vi "Actor Core.vi"(8 "error in":errorcluster, 11 "CS++DCPwrGui.lvclass":refnum<class "CS++DCPwrGui.lvclass">) -> (0 "Error Out":errorcluster, 3 "Actor out":refnum<class "Actor.lvclass">)   [LabVIEW 2014, in "CS++DCPwrGui.lvlib" / "CS++DCPwrGui.lvclass"]
doc: "(<B>Filename</B>: Actor Framework.lvlib:Actor.lvclass:Actor Core.vi)\n\nReceives messages to the actor, reacts to them, and initiates any error handling that may shut the actor down.\n\nDescendant classes may override this VI to append parallel tasks for the actor to complete while it handles messages. Overrides use the Call Parent Method node."
uses:
  CS++DCPwrGui.lvclass
  <vilib>/ActorFramework/Actor/Actor.lvclass
  CSPP_Core/Actors/CS++BaseActor/CS++BaseActor.lvclass/CS++BaseActor.ctl
  CS++DCPwrChannelData/CS++DCPwrChannelData.lvclass
  CSPP_Core/Actors/CS++GUIActor/CS++GUIActor.lvclass/CS++GUIActor.ctl
  <vilib>/ActorFramework/Actor/Actor.lvclass/Actor.ctl
  <vilib>/ActorFramework/Message Enqueuer/Message Enqueuer.lvclass/Message Enqueuer.ctl
  CSPP_Core/Classes/CS++ProcessVariables/ProcessVariable/PV.lvclass/PV.ctl
  CS++DCPwrChannelData/CS++DCPwrChannelData.lvclass/CS++DCPwrChannelData.ctl
  CS++DCPwr Messages/Configure Voltage Level Msg/Configure Voltage Level Msg.lvclass/Configure Voltage Level Msg.ctl
  CS++DCPwr Messages/Reset Output Protection Msg/Reset Output Protection Msg.lvclass/Reset Output Protection Msg.ctl
  CS++DCPwr Messages/Measure [MSR] Msg/Measure [MSR] Msg.lvclass
  CS++DCPwr Messages/Measure [MSR] Msg/Measure [MSR] Msg.lvclass/Measure [MSR] Msg.ctl
  <vilib>/ActorFramework/Batch Msg/Batch Msg.lvclass/Batch Msg.ctl
  CS++DCPwr Messages/Configure Output Enable Msg/Configure Output Enable Msg.lvclass/Configure Output Enable Msg.ctl
  CS++DCPwr Messages/Configure Desired Output State Msg/Configure Desired Output State Msg.lvclass/Configure Desired Output State Msg.ctl
  CS++DCPwr Messages/Configure Output Range Msg/Configure Output Range Msg.lvclass/Configure Output Range Msg.ctl
  CS++DCPwr Messages/Configure OVP Msg/Configure OVP Msg.lvclass/Configure OVP Msg.ctl
  CS++DCPwr Messages/Configure Current Limit Msg/Configure Current Limit Msg.lvclass/Configure Current Limit Msg.ctl
  CS++DCPwr Messages/Configure Trigger Source [TRG] Msg/Configure Trigger Source [TRG] Msg.lvclass/Configure Trigger Source [TRG] Msg.ctl
  CS++DCPwr Messages/Configure Triggered Current Limit [TRG] Msg/Configure Triggered Current Limit [TRG] Msg.lvclass/Configure Triggered Current Limit [TRG] Msg.ctl
  CS++DCPwr Messages/Configure Triggered Voltage Level [TRG] Msg/Configure Triggered Voltage Level [TRG] Msg.lvclass/Configure Triggered Voltage Level [TRG] Msg.ctl
  CSPP_Core/Actors/CS++BaseActor/Read Object Name.vi
  CSPP_Core/Actors/CS++BaseActor/Read CS++Factory.vi
  CSPP_Core/Classes/CS++ProcessVariables/ProcessVariable/Read Data.vi
  CSPP_Core/Classes/CS++ProcessVariables/ProcessVariable/Read Timestamp.vi
  CSPP_Core/Classes/CS++ProcessVariables/ProcessVariable/Read Name.vi
  CS++DCPwr Messages/Measure [MSR] Msg/Write channel name.vi
  CS++DCPwr Messages/Measure [MSR] Msg/Write measurement type.vi
  <vilib>/ActorFramework/Message Enqueuer/Init from Existing Queue.vi
  <vilib>/ActorFramework/Message Enqueuer/Enqueue.vi
  CSPP_Core/Actors/CS++GUIActor/Read Associated Actor Name.vi
  <vilib>/ActorFramework/Message Priority Queue/Priority Enqueue.vi
  CSPP_Core/Classes/CS++BaseClasses/Factory/CS++Factory.lvclass
  CSPP_Core/Classes/CS++ProcessVariables/ProcessVariable/PV.lvclass
  <vilib>/ActorFramework/Message Enqueuer/Message Enqueuer.lvclass
  <vilib>/ActorFramework/Stop Msg/Stop Msg.lvclass
  CS++DCPwr Messages/Configure Voltage Level Msg/Configure Voltage Level Msg.lvclass
  CS++DCPwr Messages/Reset Output Protection Msg/Reset Output Protection Msg.lvclass
  CS++DCPwr Messages/Initiate [TRG] Msg/Initiate [TRG] Msg.lvclass
  CS++DCPwr Messages/Send Software Trigger [SWT] Msg/Send Software Trigger [SWT] Msg.lvclass
  CS++DCPwr Messages/Abort [TRG] Msg/Abort [TRG] Msg.lvclass
  <vilib>/ActorFramework/Batch Msg/Batch Msg.lvclass
  CS++DCPwr Messages/Configure Output Enable Msg/Configure Output Enable Msg.lvclass
  CS++DCPwr Messages/Configure Desired Output State Msg/Configure Desired Output State Msg.lvclass
  CS++DCPwr Messages/Configure Output Range Msg/Configure Output Range Msg.lvclass
  CS++DCPwr Messages/Configure OVP Msg/Configure OVP Msg.lvclass
  CS++DCPwr Messages/Configure Current Limit Msg/Configure Current Limit Msg.lvclass
  CS++DCPwr Messages/Configure Trigger Source [TRG] Msg/Configure Trigger Source [TRG] Msg.lvclass
  CS++DCPwr Messages/Configure Triggered Current Limit [TRG] Msg/Configure Triggered Current Limit [TRG] Msg.lvclass
  CS++DCPwr Messages/Configure Triggered Voltage Level [TRG] Msg/Configure Triggered Voltage Level [TRG] Msg.lvclass
  CSPP_Core/Actors/CS++DeviceGUIActor/CS++DeviceGUIActor.lvclass
  CSPP_Core/Actors/CS++BaseActor/CS++BaseActor.lvclass
  CSPP_Core/Actors/CS++GUIActor/CS++GUIActor.lvclass
  CSPP_Core/Libraries/Utilities/CS++Utilities.lvlib
panel:
  in  "Tab Control":enum32{"Info", "Configuration", "Output"}(tab)
  out "Associated Actor":string
  out "Driver Revision":string
  out "Firmware Revision":string
  out "Self-Test Result Code":i32
  out "Self-Test Result Message":string
  out "Resource Name":string
  out "Number Of Channels":i32
  in  "Config Index":i32 min=0 step=1
  in  "OVP":T1 {"OVP Limit" format="%^.3g"}
  in  "Current":T2 {"Behavior" items=["Regulate", "Trip"]; "Current Limit" format="%^.3g"}
  in  "Range":cluster{"Range Type":i32, "Range":dbl}={"Range Type"=1, "Range"=0.0} {"Range" format="%^.3g"; "Range Type" items=["Voltage"=1, "Current"=0]}
  in  "Output State":i32(ring) caption="output state (Constant Voltage)" items=["Constant Voltage"=0, "Constant Current"=1, "Unregulated"=4, "Over Voltage"=2, "Over Current"=3]
  in  "Output Enable":bool caption="enabled (true)"
  in  "Trigger":T3 {"Triggered I-Limit" format="%^.6g"; "Triggered U-Level" format="%^.6g"; "Trigger Source" items=["Immediate", "External", "Software", "TTL0", "TTL1", "TTL2", "TTL3", "TTL4", "TTL5", "TTL6", "TTL7", "ECL0", "ECL1", "PXI Star", "RTSI 0", "RTSI 1", "RTSI 2", "RTSI 3", "RTSI 4", "RTSI 5", "RTSI 6"]}
  out "Maximum Limits":T4 {"Max Voltage Level" format="%^.3g"; "Max Current Limit" format="%^.3g"}
  in  "Level":dbl[unit] caption="level (0.0 Volts)" format="%^.6g"
  in  "Channel Index":i32 min=0 step=1
  in  "Reset Output Protection":bool
  in  "Initiate":bool
  in  "Software Trigger":bool
  in  "Abort":bool
  in  "Sense now":bool
  out "Timestamp":timestamp
  out "Measurements":T5(array[cluster]) {"Actual U" format="%.6g"; "Actual I" format="%.6g"}
  in  "Stop Button":bool
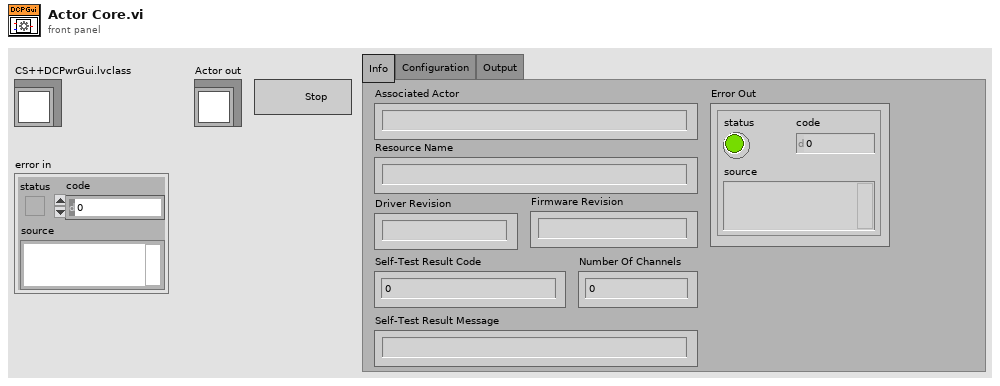
[diagram p1: front panel]
types:
  T1 = cluster{"OVP Enabled":bool, "OVP Limit":dbl[unit]}
  T2 = cluster{"Behavior":i32, "Current Limit":dbl[unit]}
  T3 = cluster{"Trigger Source":i32, "Triggered U-Level":dbl[unit], "Triggered I-Limit":dbl[unit]}
  T4 = cluster{"Max Current Limit":dbl[unit], "Max Voltage Level":dbl[unit]}
  T5 = cluster{"Actual U":dbl[unit], "Actual I":dbl[unit], "In State":bool}[]
  T6 = enum32{"Invalid", "Standard", "Closed", "Hidden", "Minimized", "Maximized"}
  T7 = cluster{"measurement":dbl[unit], "measurement":dbl[unit], "in state":bool}[]
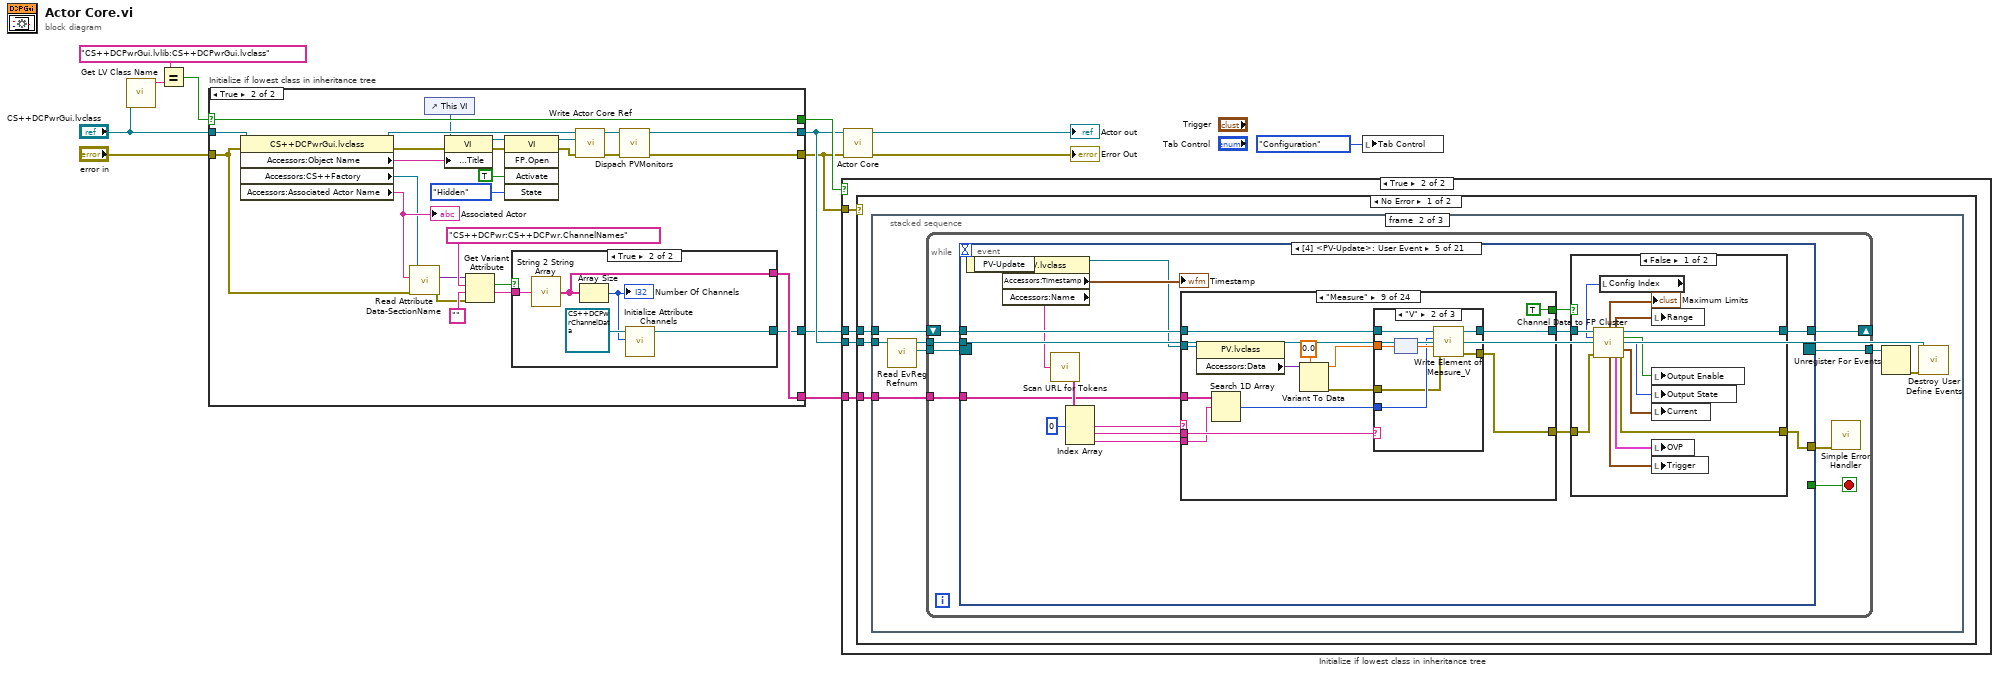
[diagram p0: block diagram]
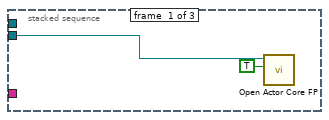
[diagram p5: hidden frame]
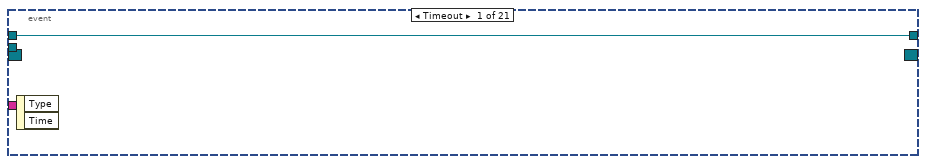
[diagram p6: hidden frame]
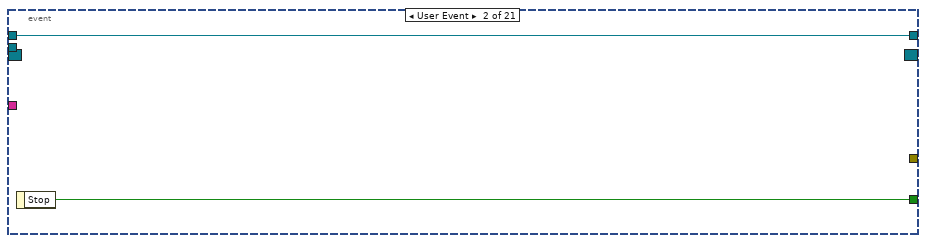
[diagram p7: hidden frame]
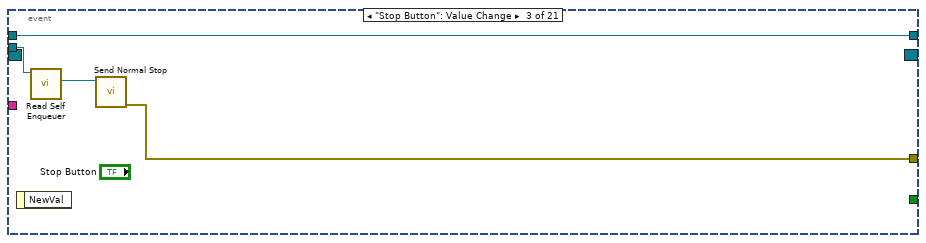
[diagram p8: hidden frame]
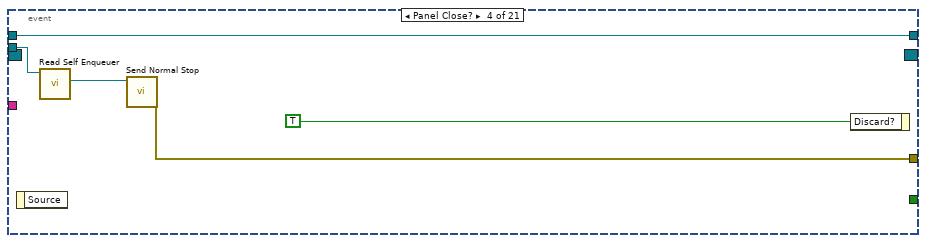
[diagram p9: hidden frame]
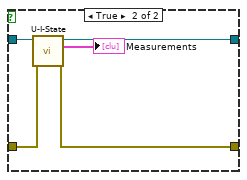
[diagram p10: hidden frame]
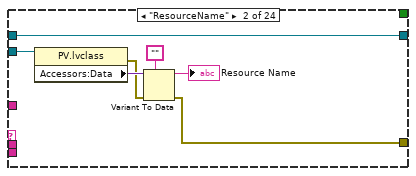
[diagram p12: hidden frame]
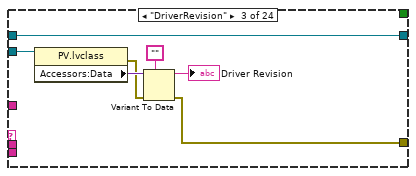
[diagram p13: hidden frame]
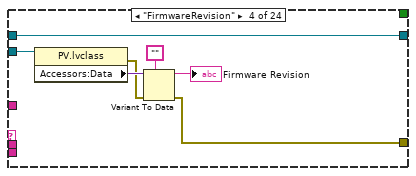
[diagram p14: hidden frame]
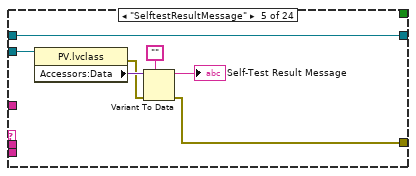
[diagram p15: hidden frame]
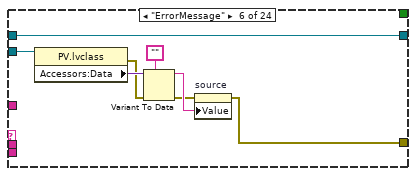
[diagram p16: hidden frame]
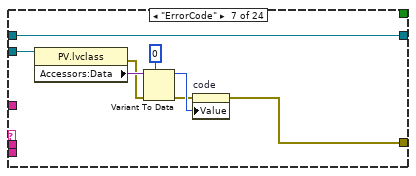
[diagram p17: hidden frame]
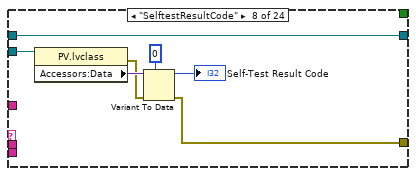
[diagram p18: hidden frame]
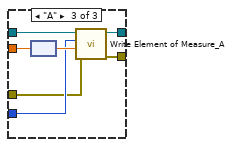
[diagram p20: hidden frame]
diagram:
  n1 = call <vilib>:"Get LV Class Name.vi"("object"="CS++DCPwrGui.lvclass") -> ("class name"=w11:string)  [unwired: 9 in, 1 out]
  n2 = Equal?(x="CS++DCPwrGui.lvlib:CS++DCPwrGui.lvclass" ("class name"), y=w11) -> (x = y?=w9:bool)
  n3 = case "Initialize if lowest class in inheritance tree" shown="True" w9 {
    selector: w9 -> [w14 w43]
    tunnel: [w15 w22] -> w4
    tunnel: "error in" -> [w15 w21]
    tunnel: [w16 w23] -> w5
    tunnel: "CS++DCPwrGui.lvclass" -> [w16 w24]
    tunnel: [w14 w43] -> w8
    tunnel: [_ w38] -> w2
    tunnel: [_ w37] -> w1
    frame False {
    }
    frame True {
      n4 = property class="CS++DCPwrGui.lvclass"(reference=w24, error in=w21) -> (reference out=w33:refnum<class "CS++DCPwrGui.lvclass">, error out=w32:errorcluster, "Accessors:Object Name"=w34:string, "Accessors:CS++Factory"=w19:refnum<class "CS++Factory.lvclass">, "Accessors:Associated Actor Name"=w20:string)
      "Associated Actor" <- w20
      n5 = call-dynamic "Read Attribute Data-SectionName.vi"("error in (no error)"=w21, "Object Name"=w20, "CS++Factory in"=w19) -> ("error out"=w17:errorcluster, "Attribute Data"=w18:variant)  [unwired: 6 in, 1 out]
      n6 = control-ref of="This VI"() -> (w29:refnum<vi>)
      n7 = property class="VI"(reference=w29, error in=w32, "Front Panel.Title"=w34) -> (reference out=w30:refnum<vi>, error out=w31:errorcluster)
      n8 = Get Variant Attribute(Variant=w18, name="CS++DCPwr:CS++DCPwr.ChannelNames", default value (empty Variant)="", error in=w17) -> (found=w40:bool, value=w39:string)  [unwired: 2 out]
      n9 = invoke class="VI" method="FP.Open"(reference=w30, error in=w31, "Activate"=TRUE ("Activate?"), "State"=T6."Hidden") -> (reference out=w27:refnum<vi>, error out=w28:errorcluster)  [unwired: 1 in, 3 out]
      n10 = case shown="True" w40 {
        tunnel: w39 -> [_ w44]
        tunnel: [_ w45] -> w38
        tunnel: [_ w46] -> w37
        frame False {
        }
        frame True {
          n11 = call "String 2 String Array.vi"("String"=w44) -> ("Substrings"=w45:string[])  [unwired: 1 in]
          n12 = Array Size(array=w45) -> (size(s)=w47:i32)
          "Number Of Channels" <- w47
          n13 = call "Initialize Attribute Channels.vi"("Number of Channels"=w47, "CS++DCPwrChannelData in"=refnum<class "CS++DCPwrChannelData.lvclass"> refnum ("CS++DCPwrGui.lvlib:CS++DCPwrChannelData.lvclass")) -> ("CS++DCPwrChannelData out"=w46:refnum<class "CS++DCPwrChannelData.lvclass">)  [unwired: 8 in, 1 out]
        }
      }
      n14 = call "Write Actor Core Ref.vi"("error in (no error)"=w28, "Actor Core Ref"=w27, "CS++BaseActor in"=w33) -> ("error out"=w36:errorcluster, "CS++BaseActor out"=w35:refnum<class "CS++DCPwrGui.lvclass">)  [unwired: 7 in]
      n15 = call "Dispach PVMonitors.vi"("Error In"=w36, "CS++GUIActor in"=w35) -> ("Error Out"=w22:errorcluster, "CS++GUIActor out"=w23:refnum<class "CS++DCPwrGui.lvclass">)  [unwired: 8 in]
    }
  }
  n16 = case "Initialize if lowest class in inheritance tree" shown="True" w8 {
    tunnel: w4 -> [_ w52]
    tunnel: w5 -> [_ w51]
    tunnel: w2 -> [_ w50]
    tunnel: w1 -> [_ w49]
    frame False {
    }
    frame True {
      n17 = case shown="No Error" w52 {
        tunnel: w51 -> [w55 _]
        tunnel: w50 -> [w54 _]
        tunnel: w49 -> [w53 _]
        frame No Error {
          n18 = stacked-sequence {
            tunnel: w55 -> [w57 w61 w522]
            tunnel: w54 -> [_ w64 _]
            tunnel: w53 -> [_ w63 _]
            frame #0 {
              n19 = call "Open Actor Core FP.vi"("Open FP (F)"=TRUE, "CS++BaseActor in"=w57) -> ()  [unwired: 8 in, 2 out]
            }
            frame #1 {
              n20 = call "Read EvReg Refnum.vi"("CS++GUIActor in"=w61) -> ("EvReg Refnum"=w60:refnum<event-registration>, "CS++GUIActor out"=w58:refnum<class "CS++DCPwrGui.lvclass">)  [unwired: 8 in, 1 out]
              n21 = while {
                tunnel: w58 -> [w72]
                tunnel: [w70] -> w62
                tunnel: w64 -> [w68]
                shift-right: [w66] -> _
                shift-left: w63 -> [w67]
                tunnel: w60 -> [w65]
                stop <- w71 stop-if-true
                n22 = event shown="[4] <PV-Update>: User Event" {
                  selector: w65 -> [_ _ _ _ _ _ _ _ _ _ _ _ _ _ _ _ _ _ _ _ _]
                  dyn-events: [_ _ _ _ _ _ _ _ _ _ _ _ _ _ _ _ _ _ _ _ _] -> w70
                  timeout: _ -> [_ _ _ _ _ _ _ _ _ _ _ _ _ _ _ _ _ _ _ _ _]
                  tunnel: w72 -> [_ _ w79 w82 _ _ w383 w408 w415 w419 w423 w432 _ w457 w465 w475 w485 w495 w503 w511 w519]
                  tunnel: [_ w75 _ _ _ _ _ _ _ _ _ _ _ _ _ _ _ _ _ _ _] -> w71
                  tunnel: [_ _ w77 w81 w89 _ w380 w406 w413 w417 w421 w425 _ w451 w459 w472 w482 w492 w497 w505 w513] -> w69
                  tunnel: w68 -> [_ _ _ _ w92 _ w379 w402 _ _ _ w430 _ w454 w464 w474 w483 w494 w501 w509 w517]
                  tunnel: w67 -> [w73 w74 w76 w80 w94 w376 w377 w399 w412 w416 w420 w424 w443 w458 w466 w476 w486 w496 w504 w512 w520]
                  tunnel: [w73 w74 w76 w80 w91 w373 w377 w399 w412 w416 w420 w424 w442 w458 w466 w476 w486 w496 w504 w512 w520] -> w66
                  event Timeout {
                    n23 = event-data() -> ()  [unwired: 1 in, 2 out]
                  }
                  event User Event {
                    n24 = event-data() -> ("Stop"=w75:bool)  [unwired: 1 in]
                  }
                  event "Stop Button": Value Change {
                    n25 = event-data() -> ()  [unwired: 1 in, 1 out]
                    n26 = call <vilib>:"Read Self Enqueuer.vi"("Actor"=w79) -> ("Self Enqueuer"=w78:refnum<class "Message Enqueuer.lvclass">)  [unwired: 10 in]
                    n27 = call <vilib>:"Send Normal Stop.vi"("Message Enqueuer"=w78) -> ("error out"=w77:errorcluster)  [unwired: 10 in]
                  }
                  event Panel Close? {
                    n28 = event-data() -> ()  [unwired: 1 in, 1 out]
                    n29 = call <vilib>:"Read Self Enqueuer.vi"("Actor"=w82) -> ("Self Enqueuer"=w83:refnum<class "Message Enqueuer.lvclass">)  [unwired: 10 in]
                    n30 = call <vilib>:"Send Normal Stop.vi"("Message Enqueuer"=w83) -> ("error out"=w81:errorcluster)  [unwired: 10 in]
                    n31 = event-data("Discard?"=TRUE) -> ()  [unwired: 1 in, 1 out]
                  }
                  event User Event {
                    n32 = event-data() -> ("PV-Update"=w96:refnum<class "PV.lvclass">)  [unwired: 1 in]
                    n33 = property class="PV.lvclass"(reference=w96) -> (reference out=w87:refnum<class "PV.lvclass">, "Accessors:Timestamp"=→"Timestamp":timestamp, "Accessors:Name"=w85:string)  [unwired: 1 in, 1 out]
                    n34 = call "Scan URL for Tokens.vi"("URL"=w85) -> ("Tokens"=w100:string[])
                    n35 = Index Array(array=w100, index #1=0 ("index")) -> (element #1=w86:string, element #2=w98:string, element #3=w97:string)  [unwired: 2 in]
                    n36 = case shown="\"Measure\"" w86 {
                      tunnel: w87 -> [_ w124 w131 w138 w145 w153 w161 w168 w180 w207 w218 w229 w240 w251 w263 w274 w286 w296 w307 w319 w331 w343 w355 w369]
                      tunnel: w98 -> [_ _ _ _ _ _ _ _ w177 w200 w211 w227 w233 w244 w255 w267 w278 w290 w300 w311 w323 w335 w347 w359]
                      tunnel: w97 -> [_ _ _ _ _ _ _ _ w172 _ _ _ _ _ _ _ _ _ _ _ _ _ _ _]
                      tunnel: w94 -> [w118 w123 w130 w137 w144 w152 w160 w167 w179 w206 w217 w226 w239 w250 w262 w273 w285 w295 w306 w318 w330 w342 w354 w365]
                      tunnel: [w118 w123 w130 w137 w144 w152 w160 w167 w178 w205 w213 w225 w238 w249 w261 w272 w284 w294 w305 w317 w329 w341 w353 w363] -> w93
                      tunnel: [_ w122 w129 w136 w143 w147 w155 w166 w175 w202 w214 w224 w235 w246 w257 w270 w283 w293 w304 w315 w328 w340 w352 w361] -> w90
                      tunnel: w92 -> [_ _ _ _ _ _ _ _ w173 w201 w212 w228 w234 w245 w256 w268 w279 w291 w301 w312 w324 w336 w348 w360]
                      tunnel: [_ _ _ _ _ _ _ _ TRUE TRUE _ _ _ _ _ _ _ _ _ _ _ _ _ _] -> w88
                      frame Default {
                      }
                      frame "ResourceName" {
                        n37 = property class="PV.lvclass"(reference=w124) -> (error out=w120:errorcluster, "Accessors:Data"=w125:variant)  [unwired: 1 in, 1 out]
                        n38 = Variant To Data(error in=w120, type="", Variant=w125) -> (data=→"Resource Name":string, error out=w122:errorcluster)
                      }
                      frame "DriverRevision" {
                        n39 = property class="PV.lvclass"(reference=w131) -> (error out=w127:errorcluster, "Accessors:Data"=w132:variant)  [unwired: 1 in, 1 out]
                        n40 = Variant To Data(error in=w127, type="", Variant=w132) -> (data=→"Driver Revision":string, error out=w129:errorcluster)
                      }
                      frame "FirmwareRevision" {
                        n41 = property class="PV.lvclass"(reference=w138) -> (error out=w134:errorcluster, "Accessors:Data"=w139:variant)  [unwired: 1 in, 1 out]
                        n42 = Variant To Data(error in=w134, type="", Variant=w139) -> (data=→"Firmware Revision":string, error out=w136:errorcluster)
                      }
                      frame "SelftestResultMessage" {
                        n43 = property class="PV.lvclass"(reference=w145) -> (error out=w141:errorcluster, "Accessors:Data"=w146:variant)  [unwired: 1 in, 1 out]
                        n44 = Variant To Data(error in=w141, type="", Variant=w146) -> (data=→"Self-Test Result Message":string, error out=w143:errorcluster)
                      }
                      frame "ErrorMessage" {
                        n45 = property class="PV.lvclass"(reference=w153) -> (error out=w150:errorcluster, "Accessors:Data"=w154:variant)  [unwired: 1 in, 1 out]
                        n46 = Variant To Data(error in=w150, type="", Variant=w154) -> (data=w149:string, error out=w148:errorcluster)
                        n47 = property on="source" class="Str"(error in=w148, "Value"=w149) -> (error out=w147:errorcluster)  [unwired: 1 in, 1 out]
                      }
                      frame "ErrorCode" {
                        n48 = property class="PV.lvclass"(reference=w161) -> (error out=w158:errorcluster, "Accessors:Data"=w162:variant)  [unwired: 1 in, 1 out]
                        n49 = Variant To Data(error in=w158, type=0, Variant=w162) -> (data=w157:i32, error out=w156:errorcluster)
                        n50 = property on="code" class="DigNum (strict)"(error in=w156, "Value"=w157) -> (error out=w155:errorcluster)  [unwired: 1 in, 1 out]
                      }
                      frame "SelftestResultCode" {
                        n51 = property class="PV.lvclass"(reference=w168) -> (error out=w164:errorcluster, "Accessors:Data"=w169:variant)  [unwired: 1 in, 1 out]
                        n52 = Variant To Data(error in=w164, type=0, Variant=w169) -> (data=→"Self-Test Result Code":i32, error out=w166:errorcluster)
                      }
                      frame "Measure" {
                        n53 = property class="PV.lvclass"(reference=w180) -> ("Accessors:Data"=w181:variant)  [unwired: 1 in, 2 out]
                        n54 = Search 1D Array(1D array=w173, element=w172) -> (index of element=w171:i32)  [unwired: 1 in]
                        n55 = Variant To Data(type=0.0, Variant=w181) -> (data=w176:dbl, error out=w174:errorcluster)  [unwired: 1 in]
                        n56 = case shown="\"V\"" w177 {
                          tunnel: w179 -> [w183 w190 w196]
                          tunnel: [w183 w189 w195] -> w178
                          tunnel: w176 -> [_ w187 w197]
                          tunnel: w171 -> [_ w186 w193]
                          tunnel: [_ w185 w192] -> w175
                          tunnel: w174 -> [_ w184 w191]
                          frame Default {
                          }
                          frame "V" {
                            n57 = node(w187) -> (w188:dbl[unit])
                            n58 = call "Write Element of Measure_V.vi"("error in (no error)"=w184, "measurement"=w188, "index"=w186, "CS++DCPwrChannelData in"=w190) -> ("error out"=w185:errorcluster, "CS++DCPwrChannelData out"=w189:refnum<class "CS++DCPwrChannelData.lvclass">)  [unwired: 6 in]
                          }
                          frame "A" {
                            n59 = node(w197) -> (w194:dbl[unit])
                            n60 = call "Write Element of Measure_A.vi"("error in (no error)"=w191, "measurement"=w194, "index"=w193, "CS++DCPwrChannelData in"=w196) -> ("error out"=w192:errorcluster, "CS++DCPwrChannelData out"=w195:refnum<class "CS++DCPwrChannelData.lvclass">)  [unwired: 6 in]
                          }
                        }
                      }
                      frame "InState" {
                        n61 = property class="PV.lvclass"(reference=w207) -> ("Accessors:Data"=w208:variant)  [unwired: 1 in, 2 out]
                        n62 = Search 1D Array(1D array=w201, element=w200) -> (index of element=w199:i32)  [unwired: 1 in]
                        n63 = Variant To Data(type=FALSE, Variant=w208) -> (data=w204:bool, error out=w203:errorcluster)  [unwired: 1 in]
                        n64 = call "Write Element of In State.vi"("error in (no error)"=w203, "in state"=w204, "index"=w199, "CS++DCPwrChannelData in"=w206) -> ("error out"=w202:errorcluster, "CS++DCPwrChannelData out"=w205:refnum<class "CS++DCPwrChannelData.lvclass">)  [unwired: 6 in]
                      }
                      frame "OutputEnable" {
                        n65 = property class="PV.lvclass"(reference=w218) -> ("Accessors:Data"=w219:variant)  [unwired: 1 in, 2 out]
                        n66 = Search 1D Array(1D array=w212, element=w211) -> (index of element=w210:i32)  [unwired: 1 in]
                        n67 = Variant To Data(type=FALSE, Variant=w219) -> (data=w216:bool, error out=w215:errorcluster)  [unwired: 1 in]
                        n68 = call "Write Element of Output Enable.vi"("error in (no error)"=w215, "enabled (true)"=w216, "index"=w210, "CS++DCPwrChannelData in"=w217) -> ("error out"=w214:errorcluster, "CS++DCPwrChannelData out"=w213:refnum<class "CS++DCPwrChannelData.lvclass">)  [unwired: 6 in]
                      }
                      frame "DesiredOutputState" {
                        n69 = property class="PV.lvclass"(reference=w229) -> ("Accessors:Data"=w230:variant)  [unwired: 1 in, 2 out]
                        n70 = Search 1D Array(1D array=w228, element=w227) -> (index of element=w223:i32)  [unwired: 1 in]
                        n71 = Variant To Data(type=0, Variant=w230) -> (data=w222:i32, error out=w221:errorcluster)  [unwired: 1 in]
                        n72 = call "Write Element of Desired Output State.vi"("error in (no error)"=w221, "output state (Constant Voltage)"=w222, "index"=w223, "CS++DCPwrChannelData in"=w226) -> ("error out"=w224:errorcluster, "CS++DCPwrChannelData out"=w225:refnum<class "CS++DCPwrChannelData.lvclass">)  [unwired: 6 in]
                      }
                      frame "RangeType" {
                        n73 = property class="PV.lvclass"(reference=w240) -> ("Accessors:Data"=w241:variant)  [unwired: 1 in, 2 out]
                        n74 = Search 1D Array(1D array=w234, element=w233) -> (index of element=w232:i32)  [unwired: 1 in]
                        n75 = Variant To Data(type=0, Variant=w241) -> (data=w237:i32, error out=w236:errorcluster)  [unwired: 1 in]
                        n76 = call "Write Element of Range Type.vi"("error in (no error)"=w236, "range type (Voltage)"=w237, "index"=w232, "CS++DCPwrChannelData in"=w239) -> ("error out"=w235:errorcluster, "CS++DCPwrChannelData out"=w238:refnum<class "CS++DCPwrChannelData.lvclass">)  [unwired: 6 in]
                      }
                      frame "Range" {
                        n77 = property class="PV.lvclass"(reference=w251) -> ("Accessors:Data"=w252:variant)  [unwired: 1 in, 2 out]
                        n78 = Search 1D Array(1D array=w245, element=w244) -> (index of element=w243:i32)  [unwired: 1 in]
                        n79 = Variant To Data(type=0.0, Variant=w252) -> (data=w248:dbl, error out=w247:errorcluster)  [unwired: 1 in]
                        n80 = call "Write Element of Range.vi"("error in (no error)"=w247, "range (0.0)"=w248, "index"=w243, "CS++DCPwrChannelData in"=w250) -> ("error out"=w246:errorcluster, "CS++DCPwrChannelData out"=w249:refnum<class "CS++DCPwrChannelData.lvclass">)  [unwired: 6 in]
                      }
                      frame "CurrentLimit" {
                        n81 = property class="PV.lvclass"(reference=w263) -> ("Accessors:Data"=w264:variant)  [unwired: 1 in, 2 out]
                        n82 = Search 1D Array(1D array=w256, element=w255) -> (index of element=w254:i32)  [unwired: 1 in]
                        n83 = Variant To Data(type=0.0, Variant=w264) -> (data=w259:dbl, error out=w260:errorcluster)  [unwired: 1 in]
                        n84 = node(w259) -> (w258:dbl[unit])
                        n85 = call "Write Element of Current Limit.vi"("error in (no error)"=w260, "limit (0.0 Amps)"=w258, "index"=w254, "CS++DCPwrChannelData in"=w262) -> ("error out"=w257:errorcluster, "CS++DCPwrChannelData out"=w261:refnum<class "CS++DCPwrChannelData.lvclass">)  [unwired: 6 in]
                      }
                      frame "Behavior" {
                        n86 = property class="PV.lvclass"(reference=w274) -> ("Accessors:Data"=w275:variant)  [unwired: 1 in, 2 out]
                        n87 = Search 1D Array(1D array=w268, element=w267) -> (index of element=w266:i32)  [unwired: 1 in]
                        n88 = Variant To Data(type=0, Variant=w275) -> (data=w269:i32, error out=w271:errorcluster)  [unwired: 1 in]
                        n89 = call "Write Element of Behavior.vi"("error in (no error)"=w271, "behavior (regulate)"=w269, "index"=w266, "CS++DCPwrChannelData in"=w273) -> ("error out"=w270:errorcluster, "CS++DCPwrChannelData out"=w272:refnum<class "CS++DCPwrChannelData.lvclass">)  [unwired: 6 in]
                      }
                      frame "OVPLimit" {
                        n90 = property class="PV.lvclass"(reference=w286) -> ("Accessors:Data"=w287:variant)  [unwired: 1 in, 2 out]
                        n91 = Search 1D Array(1D array=w279, element=w278) -> (index of element=w277:i32)  [unwired: 1 in]
                        n92 = Variant To Data(type=0.0, Variant=w287) -> (data=w281:dbl, error out=w282:errorcluster)  [unwired: 1 in]
                        n93 = node(w281) -> (w280:dbl[unit])
                        n94 = call "Write Element of OVP Limit.vi"("error in (no error)"=w282, "limit (0.0 Volts)"=w280, "index"=w277, "CS++DCPwrChannelData in"=w285) -> ("error out"=w283:errorcluster, "CS++DCPwrChannelData out"=w284:refnum<class "CS++DCPwrChannelData.lvclass">)  [unwired: 6 in]
                      }
                      frame "OVPEnabled" {
                        n95 = property class="PV.lvclass"(reference=w296) -> ("Accessors:Data"=w297:variant)  [unwired: 1 in, 2 out]
                        n96 = Search 1D Array(1D array=w291, element=w290) -> (index of element=w289:i32)  [unwired: 1 in]
                        n97 = Variant To Data(type=FALSE, Variant=w297) -> (data=w292:bool)  [unwired: 1 in, 1 out]
                        n98 = call "Write Element of OVP Enabled.vi"("enabled (true)"=w292, "index"=w289, "CS++DCPwrChannelData in"=w295) -> ("error out"=w293:errorcluster, "CS++DCPwrChannelData out"=w294:refnum<class "CS++DCPwrChannelData.lvclass">)  [unwired: 7 in]
                      }
                      frame "TriggerSource" {
                        n99 = property class="PV.lvclass"(reference=w307) -> ("Accessors:Data"=w308:variant)  [unwired: 1 in, 2 out]
                        n100 = Search 1D Array(1D array=w301, element=w300) -> (index of element=w299:i32)  [unwired: 1 in]
                        n101 = Variant To Data(type=0, Variant=w308) -> (data=w302:i32, error out=w303:errorcluster)  [unwired: 1 in]
                        n102 = call "Write Element of Trigger Source.vi"("error in (no error)"=w303, "source (Immediate)"=w302, "index"=w299, "CS++DCPwrChannelData in"=w306) -> ("error out"=w304:errorcluster, "CS++DCPwrChannelData out"=w305:refnum<class "CS++DCPwrChannelData.lvclass">)  [unwired: 6 in]
                      }
                      frame "TriggerVoltageLevel" {
                        n103 = property class="PV.lvclass"(reference=w319) -> ("Accessors:Data"=w320:variant)  [unwired: 1 in, 2 out]
                        n104 = Search 1D Array(1D array=w312, element=w311) -> (index of element=w310:i32)  [unwired: 1 in]
                        n105 = Variant To Data(type=0.0, Variant=w320) -> (data=w313:dbl, error out=w316:errorcluster)  [unwired: 1 in]
                        n106 = node(w313) -> (w314:dbl[unit])
                        n107 = call "Write Element of Trigger Voltage Level.vi"("error in (no error)"=w316, "triggered level (0.0 Volts)"=w314, "index"=w310, "CS++DCPwrChannelData in"=w318) -> ("error out"=w315:errorcluster, "CS++DCPwrChannelData out"=w317:refnum<class "CS++DCPwrChannelData.lvclass">)  [unwired: 6 in]
                      }
                      frame "TriggerCurrentLimit" {
                        n108 = property class="PV.lvclass"(reference=w331) -> ("Accessors:Data"=w332:variant)  [unwired: 1 in, 2 out]
                        n109 = Search 1D Array(1D array=w324, element=w323) -> (index of element=w322:i32)  [unwired: 1 in]
                        n110 = Variant To Data(type=0.0, Variant=w332) -> (data=w326:dbl, error out=w327:errorcluster)  [unwired: 1 in]
                        n111 = node(w326) -> (w325:dbl[unit])
                        n112 = call "Write Element of Trigger Current Limit.vi"("error in (no error)"=w327, "triggered limit (0.0 Amps)"=w325, "index"=w322, "CS++DCPwrChannelData in"=w330) -> ("error out"=w328:errorcluster, "CS++DCPwrChannelData out"=w329:refnum<class "CS++DCPwrChannelData.lvclass">)  [unwired: 6 in]
                      }
                      frame "MaxVoltageLevel" {
                        n113 = property class="PV.lvclass"(reference=w343) -> ("Accessors:Data"=w344:variant)  [unwired: 1 in, 2 out]
                        n114 = Search 1D Array(1D array=w336, element=w335) -> (index of element=w334:i32)  [unwired: 1 in]
                        n115 = Variant To Data(type=0.0, Variant=w344) -> (data=w338:dbl, error out=w339:errorcluster)  [unwired: 1 in]
                        n116 = node(w338) -> (w337:dbl[unit])
                        n117 = call "Write Element of Max Voltage Level.vi"("error in (no error)"=w339, "max voltage level"=w337, "index"=w334, "CS++DCPwrChannelData in"=w342) -> ("error out"=w340:errorcluster, "CS++DCPwrChannelData out"=w341:refnum<class "CS++DCPwrChannelData.lvclass">)  [unwired: 6 in]
                      }
                      frame "MaxCurrentLimit" {
                        n118 = property class="PV.lvclass"(reference=w355) -> ("Accessors:Data"=w356:variant)  [unwired: 1 in, 2 out]
                        n119 = Search 1D Array(1D array=w348, element=w347) -> (index of element=w346:i32)  [unwired: 1 in]
                        n120 = Variant To Data(type=0.0, Variant=w356) -> (data=w349:dbl, error out=w351:errorcluster)  [unwired: 1 in]
                        n121 = node(w349) -> (w350:dbl[unit])
                        n122 = call "Write Element of Max Current Limit.vi"("error in (no error)"=w351, "max current limit"=w350, "index"=w346, "CS++DCPwrChannelData in"=w354) -> ("error out"=w352:errorcluster, "CS++DCPwrChannelData out"=w353:refnum<class "CS++DCPwrChannelData.lvclass">)  [unwired: 6 in]
                      }
                      frame "VoltageLevel" {
                        n123 = property class="PV.lvclass"(reference=w369) -> ("Accessors:Data"=w370:variant)  [unwired: 1 in, 2 out]
                        n124 = Search 1D Array(1D array=w360, element=w359) -> (index of element=w358:i32)  [unwired: 1 in]
                        n125 = local read "Channel Index"() -> (w368:i32)
                        n126 = Variant To Data(type=0.0, Variant=w370) -> (data=w366:dbl, error out=w362:errorcluster)  [unwired: 1 in]
                        n127 = node(w366) -> (w364:dbl[unit])
                        n128 = Equal?(x=w368, y=w358) -> (x = y?=w367:bool)
                        n129 = call "Write Element of Voltage Level.vi"("error in (no error)"=w362, "level (0.0 Volts)"=w364, "index"=w358, "CS++DCPwrChannelData in"=w365) -> ("error out"=w361:errorcluster, "CS++DCPwrChannelData out"=w363:refnum<class "CS++DCPwrChannelData.lvclass">)  [unwired: 6 in]
                        n130 = case shown="True" w367 {
                          tunnel: w364 -> [_ w372]
                          frame False {
                          }
                          frame True {
                            n131 = local write "Level"(w372) -> ()
                          }
                        }
                      }
                    }
                    n132 = case shown="False" w88 {
                      tunnel: w93 -> [w112 w116]
                      tunnel: [w103 w115] -> w91
                      tunnel: w90 -> [w102 w113]
                      tunnel: [w101 w114] -> w89
                      frame False {
                        n133 = local read "Config Index"() -> (w111:i32)
                        n134 = call "Channel Data to FP Cluster.vi"("CS++DCPwrChannelData in"=w112, "Channel Index"=w111, "Error In"=w102) -> ("Maximum Limits"=→"Maximum Limits":T4, "Range"=w105:cluster{"Range Type":i32, "Range":dbl}, "CS++DCPwrChannelData out"=w103:refnum<class "CS++DCPwrChannelData.lvclass">, "Output Enable"=w110:bool, "Output State"=w109:i32, "Current"=w104:T2, "Trigger"=w107:T3, "OVP"=w108:T1, "Error Out"=w101:errorcluster)  [unwired: 4 in]
                        n135 = local write "Range"(w105) -> ()
                        n136 = local write "Output Enable"(w110) -> ()
                        n137 = local write "Output State"(w109) -> ()
                        n138 = local write "Current"(w104) -> ()
                        n139 = local write "OVP"(w108) -> ()
                        n140 = local write "Trigger"(w107) -> ()
                      }
                      frame True {
                        n141 = call "U-I-State.vi"("error in (no error)"=w113, "CS++DCPwrChannelData in"=w116) -> ("error out"=w114:errorcluster, "Actual Measurements"=→"Measurements":T7, "CS++DCPwrChannelData out"=w115:refnum<class "CS++DCPwrChannelData.lvclass">)  [unwired: 7 in]
                      }
                    }
                  }
                  event "Channel Index": Value Change {
                    n142 = event-data() -> ("NewVal"=w374:i32)  [unwired: 1 in]
                    n143 = call "Read Element of Voltage Level.vi"("index"=w374, "CS++DCPwrChannelData in"=w376) -> ("level (0.0 Volts)"=w375:dbl[unit], "CS++DCPwrChannelData out"=w373:refnum<class "CS++DCPwrChannelData.lvclass">)  [unwired: 7 in, 1 out]
                    n144 = local write "Level"(w375) -> ()
                  }
                  event "Level": Value Change {
                    n145 = event-data() -> ("NewVal"=w381:dbl[unit])  [unwired: 1 in]
                    n146 = call "Read Associated Actor Enqueuer.vi"("CS++GUIActor in"=w383) -> ("Associated Actor Enqueuer"=w382:refnum<class "Message Enqueuer.lvclass">)  [unwired: 8 in, 2 out]
                    n147 = local read "Channel Index"() -> (w378:i32)
                    n148 = case shown="0.." w378 {
                      selector: w378 -> [_ w384 _]
                      tunnel: w382 -> [_ w389 w394]
                      tunnel: w381 -> [_ w388 w393]
                      tunnel: [_ w387 w390] -> w380
                      tunnel: w379 -> [_ w386 w391]
                      frame Default {
                      }
                      frame 0.. {
                        n149 = Index Array(array=w386, index=w384) -> (element=w385:string)
                        n150 = call "Send Configure Voltage Level.vi"("level (0.0 Volts)"=w388, "channel name (\"CHANNEL1\")"=w385, "Message Enqueuer"=w389) -> ("error out"=w387:errorcluster)  [unwired: 7 in, 1 out]
                      }
                      frame -2 {
                        n151 = for {
                          tunnel: w394 -> [w398]
                          tunnel: w393 -> [w397]
                          tunnel: [w396] -> w392 mode=indexing
                          tunnel: w391 -> [w395] mode=indexing
                          n152 = call "Send Configure Voltage Level.vi"("level (0.0 Volts)"=w397, "channel name (\"CHANNEL1\")"=w395, "Message Enqueuer"=w398) -> ("error out"=w396:errorcluster)  [unwired: 7 in, 1 out]
                        }
                        n153 = Merge Errors(w392) -> (w390:errorcluster)
                      }
                    }
                  }
                  event "Reset Output Protection": Value Change {
                    n154 = event-data() -> ()  [unwired: 1 in, 1 out]
                    n155 = call "Read Associated Actor Enqueuer.vi"("CS++GUIActor in"=w408) -> ("Associated Actor Enqueuer"=w407:refnum<class "Message Enqueuer.lvclass">)  [unwired: 8 in, 2 out]
                    n156 = Index Array(array=w402, index="Channel Index") -> (element=w401:string)
                    n157 = Concatenate Strings("Do you really want to reset the output protection of channel: " ("message"), w401) -> (w404:string)
                    n158 = Two Button Dialog(message=w404) -> (T button?=w403:bool)  [unwired: 2 in]
                    n159 = case shown="True" w403 {
                      tunnel: w407 -> [_ w411]
                      tunnel: [_ w410] -> w406
                      tunnel: w401 -> [_ w409]
                      frame False {
                      }
                      frame True {
                        n160 = call "Send Reset Output Protection.vi"("channel name (\"CHANNEL1\")"=w409, "Message Enqueuer"=w411) -> ("error out"=w410:errorcluster)  [unwired: 8 in, 1 out]
                      }
                    }
                  }
                  event "Initiate": Value Change {
                    n161 = event-data() -> ()  [unwired: 1 in, 1 out]
                    n162 = call "Read Associated Actor Enqueuer.vi"("CS++GUIActor in"=w415) -> ("Associated Actor Enqueuer"=w414:refnum<class "Message Enqueuer.lvclass">)  [unwired: 8 in, 2 out]
                    n163 = call "Send Initiate [TRG].vi"("Message Enqueuer"=w414) -> ("error out"=w413:errorcluster)  [unwired: 9 in, 1 out]
                  }
                  event "Software Trigger": Value Change {
                    n164 = event-data() -> ()  [unwired: 1 in, 1 out]
                    n165 = call "Read Associated Actor Enqueuer.vi"("CS++GUIActor in"=w419) -> ("Associated Actor Enqueuer"=w418:refnum<class "Message Enqueuer.lvclass">)  [unwired: 8 in, 2 out]
                    n166 = call "Send Send Software Trigger [SWT].vi"("Message Enqueuer"=w418) -> ("error out"=w417:errorcluster)  [unwired: 9 in, 1 out]
                  }
                  event "Abort": Value Change {
                    n167 = event-data() -> ()  [unwired: 1 in, 1 out]
                    n168 = call "Read Associated Actor Enqueuer.vi"("CS++GUIActor in"=w423) -> ("Associated Actor Enqueuer"=w422:refnum<class "Message Enqueuer.lvclass">)  [unwired: 8 in, 2 out]
                    n169 = call "Send Abort [TRG].vi"("Message Enqueuer"=w422) -> ("error out"=w421:errorcluster)  [unwired: 9 in, 1 out]
                  }
                  event "Sense now": Value Change {
                    w431 = refnum<class "Measure [MSR] Msg.lvclass"> refnum ("CS++DCPwr.lvlib:Measure [MSR] Msg.lvclass")
                    n170 = event-data() -> ()  [unwired: 1 in, 1 out]
                    n171 = call "Read Associated Actor Enqueuer.vi"("CS++GUIActor in"=w432) -> ("Associated Actor Enqueuer"=w426:refnum<class "Message Enqueuer.lvclass">)  [unwired: 8 in, 2 out]
                    n172 = for "Voltages" {
                      tunnel: w431 -> [w438]
                      tunnel: w430 -> [w440] mode=indexing
                      tunnel: [w437] -> w429 mode=indexing
                      n173 = property class="Measure [MSR] Msg.lvclass"(reference=w438, "Accessors:channel name"=w440, "Accessors:measurement type"=1 ("measurement type (voltage)")) -> (reference out=w437:refnum<class "Measure [MSR] Msg.lvclass">)  [unwired: 1 in, 1 out]
                    }
                    n174 = for "Currents" {
                      tunnel: w431 -> [w434]
                      tunnel: w430 -> [w436] mode=indexing
                      tunnel: [w433] -> w428 mode=indexing
                      n175 = property class="Measure [MSR] Msg.lvclass"(reference=w434, "Accessors:channel name"=w436, "Accessors:measurement type"=0 ("measurement type (voltage)")) -> (reference out=w433:refnum<class "Measure [MSR] Msg.lvclass">)  [unwired: 1 in, 1 out]
                    }
                    n176 = Build Array (concatenate)(w429, w428) -> (w427:refnum<class "Measure [MSR] Msg.lvclass">[])
                    n177 = call <vilib>:"Send Batch.vi"("Messages Array"=w427, "Message Enqueuer"=w426) -> ("error out"=w425:errorcluster)  [unwired: 9 in]
                  }
                  event "Config Index": Value Change {
                    n178 = event-data() -> ("NewVal"=w441:i32)  [unwired: 1 in]
                    n179 = call "Channel Data to FP Cluster.vi"("CS++DCPwrChannelData in"=w443, "Channel Index"=w441) -> ("Maximum Limits"=w446:T4, "Range"=w445:cluster{"Range Type":i32, "Range":dbl}, "CS++DCPwrChannelData out"=w442:refnum<class "CS++DCPwrChannelData.lvclass">, "Output Enable"=w450:bool, "Output State"=w449:i32, "Current"=w444:T2, "Trigger"=w447:T3, "OVP"=w448:T1)  [unwired: 5 in, 1 out]
                    n180 = local write "Maximum Limits"(w446) -> ()
                    n181 = local write "Range"(w445) -> ()
                    n182 = local write "Output Enable"(w450) -> ()
                    n183 = local write "Output State"(w449) -> ()
                    n184 = local write "Current"(w444) -> ()
                    n185 = local write "OVP"(w448) -> ()
                    n186 = local write "Trigger"(w447) -> ()
                  }
                  event "Output Enable": Value Change {
                    n187 = event-data() -> ("NewVal"=w455:bool)  [unwired: 1 in]
                    n188 = local read "Config Index"() -> (w452:i32)
                    n189 = call "Read Associated Actor Enqueuer.vi"("CS++GUIActor in"=w457) -> ("Associated Actor Enqueuer"=w456:refnum<class "Message Enqueuer.lvclass">)  [unwired: 8 in, 2 out]
                    n190 = Index Array(array=w454, index=w452) -> (element=w453:string)
                    n191 = call "Send Configure Output Enable.vi"("enabled (true)"=w455, "channel name (\"CHANNEL1\")"=w453, "Message Enqueuer"=w456) -> ("error out"=w451:errorcluster)  [unwired: 7 in, 1 out]
                  }
                  event "Output State": Value Change {
                    n192 = event-data() -> ("NewVal"=w460:i32)  [unwired: 1 in]
                    n193 = local read "Config Index"() -> (w463:i32)
                    n194 = call "Read Associated Actor Enqueuer.vi"("CS++GUIActor in"=w465) -> ("Associated Actor Enqueuer"=w462:refnum<class "Message Enqueuer.lvclass">)  [unwired: 8 in, 2 out]
                    n195 = Index Array(array=w464, index=w463) -> (element=w461:string)
                    n196 = call "Send Configure Desired Output State.vi"("output state (Constant Voltage)"=w460, "channel name (\"CHANNEL1\")"=w461, "Message Enqueuer"=w462) -> ("error out"=w459:errorcluster)  [unwired: 7 in, 1 out]
                  }
                  event "Range": Value Change {
                    n197 = event-data() -> ("NewVal"=w467:cluster{"Range Type":i32, "Range":dbl})  [unwired: 1 in]
                    n198 = call "Read Associated Actor Enqueuer.vi"("CS++GUIActor in"=w475) -> ("Associated Actor Enqueuer"=w473:refnum<class "Message Enqueuer.lvclass">)  [unwired: 8 in, 2 out]
                    n199 = local read "Config Index"() -> (w471:i32)
                    n200 = Unbundle By Name(w467) -> ("Range Type"=w469:i32, "Range"=w468:dbl)
                    n201 = Index Array(array=w474, index=w471) -> (element=w470:string)
                    n202 = call "Send Configure Output Range.vi"("range (0.0)"=w468, "range type (Voltage)"=w469, "channel name (\"CHANNEL1\")"=w470, "Message Enqueuer"=w473) -> ("error out"=w472:errorcluster)  [unwired: 6 in, 1 out]
                  }
                  event "OVP": Value Change {
                    n203 = event-data() -> ("NewVal"=w477:T1)  [unwired: 1 in]
                    n204 = call "Read Associated Actor Enqueuer.vi"("CS++GUIActor in"=w485) -> ("Associated Actor Enqueuer"=w484:refnum<class "Message Enqueuer.lvclass">)  [unwired: 8 in, 2 out]
                    n205 = local read "Config Index"() -> (w481:i32)
                    n206 = Unbundle By Name(w477) -> ("OVP Limit"=w479:dbl[unit], "OVP Enabled"=w478:bool)
                    n207 = Index Array(array=w483, index=w481) -> (element=w480:string)
                    n208 = call "Send Configure OVP.vi"("enabled (true)"=w478, "limit (0.0 Volts)"=w479, "channel name (\"CHANNEL1\")"=w480, "Message Enqueuer"=w484) -> ("error out"=w482:errorcluster)  [unwired: 6 in, 1 out]
                  }
                  event "Current": Value Change {
                    n209 = event-data() -> ("NewVal"=w487:T2)  [unwired: 1 in]
                    n210 = call "Read Associated Actor Enqueuer.vi"("CS++GUIActor in"=w495) -> ("Associated Actor Enqueuer"=w493:refnum<class "Message Enqueuer.lvclass">)  [unwired: 8 in, 2 out]
                    n211 = local read "Config Index"() -> (w491:i32)
                    n212 = Unbundle By Name(w487) -> ("Behavior"=w489:i32, "Current Limit"=w488:dbl[unit])
                    n213 = Index Array(array=w494, index=w491) -> (element=w490:string)
                    n214 = call "Send Configure Current Limit.vi"("limit (0.0 Amps)"=w488, "behavior (regulate)"=w489, "channel name (\"CHANNEL1\")"=w490, "Message Enqueuer"=w493) -> ("error out"=w492:errorcluster)  [unwired: 6 in, 1 out]
                  }
                  event "Trigger.Trigger Source": Value Change {
                    n215 = event-data() -> ("NewVal"=w498:i32)  [unwired: 1 in]
                    n216 = call "Read Associated Actor Enqueuer.vi"("CS++GUIActor in"=w503) -> ("Associated Actor Enqueuer"=w500:refnum<class "Message Enqueuer.lvclass">)  [unwired: 8 in, 2 out]
                    n217 = local read "Config Index"() -> (w502:i32)
                    n218 = Index Array(array=w501, index=w502) -> (element=w499:string)
                    n219 = call "Send Configure Trigger Source [TRG].vi"("source (Immediate)"=w498, "channel name (\"CHANNEL1\")"=w499, "Message Enqueuer"=w500) -> ("error out"=w497:errorcluster)  [unwired: 7 in, 1 out]
                  }
                  event "Trigger.Triggered I-Limit": Value Change {
                    n220 = event-data() -> ("NewVal"=w506:dbl[unit])  [unwired: 1 in]
                    n221 = call "Read Associated Actor Enqueuer.vi"("CS++GUIActor in"=w511) -> ("Associated Actor Enqueuer"=w508:refnum<class "Message Enqueuer.lvclass">)  [unwired: 8 in, 2 out]
                    n222 = local read "Config Index"() -> (w510:i32)
                    n223 = Index Array(array=w509, index=w510) -> (element=w507:string)
                    n224 = call "Send Configure Triggered Current Limit [TRG].vi"("triggered limit (0.0 Amps)"=w506, "channel name (\"CHANNEL1\")"=w507, "Message Enqueuer"=w508) -> ("error out"=w505:errorcluster)  [unwired: 7 in, 1 out]
                  }
                  event "Trigger.Triggered U-Level": Value Change {
                    n225 = event-data() -> ("NewVal"=w514:dbl[unit])  [unwired: 1 in]
                    n226 = call "Read Associated Actor Enqueuer.vi"("CS++GUIActor in"=w519) -> ("Associated Actor Enqueuer"=w516:refnum<class "Message Enqueuer.lvclass">)  [unwired: 8 in, 2 out]
                    n227 = local read "Config Index"() -> (w518:i32)
                    n228 = Index Array(array=w517, index=w518) -> (element=w515:string)
                    n229 = call "Send Configure Triggered Voltage Level [TRG].vi"("triggered level (0.0 Volts)"=w514, "channel name (\"CHANNEL1\")"=w515, "Message Enqueuer"=w516) -> ("error out"=w513:errorcluster)  [unwired: 7 in, 1 out]
                  }
                }
                n230 = call <vilib>:"Simple Error Handler.vi"("error in (no error)"=w69) -> ()  [unwired: 4 in, 5 out]
              }
              n231 = Unregister For Events(event registration refnum=w62) -> (error out=w59:errorcluster)  [unwired: 1 in]
              n232 = call-dynamic "Destroy User Define Events.vi"("error in (no error)"=w59, "CS++GUIActor in"=w58) -> ()  [unwired: 8 in, 2 out]
            }
            frame #2 {
              n233 = call "Open Actor Core FP.vi"("Open FP (F)"=FALSE, "CS++BaseActor in"=w522) -> ()  [unwired: 8 in, 2 out]
            }
          }
        }
        frame Error {
        }
      }
    }
  }
  n234 = call-parent "Actor Core.vi"("error in"=w4, "CS++DeviceGUIActor.lvclass"=w5) -> ("Error Out"=→"Error Out":errorcluster, "Actor out"=→"Actor out":refnum<class "Actor.lvclass">)  [unwired: 8 in]
  n235 = local write "Tab Control"(enum32{"Info", "Configuration", "Output"}."Configuration" ("Tab Control")) -> ()
